vi "FlatSequence.vi"() -> ()   [LabVIEW 2015]
panel:
  in  "stop":bool
  in  "Tab Control":enum32{"Page 1", "Page 2", "Page 3"}(tab)
  in  "Slide":dbl(slide) scale=0.0..10.0
  out "String":string="Valor de Temperatura"
  out "Slide 2":dbl(slide) scale=0.0..10.0
  out "String 2":string="Agregacion de Parametros"
  out "String 3":string="Termina Proceso"
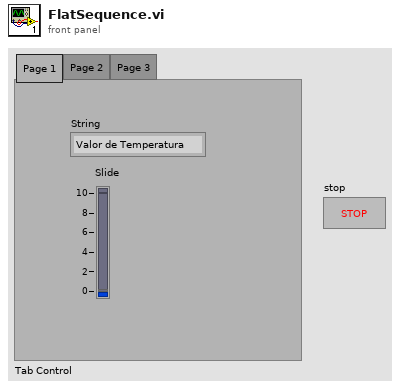
[diagram p1: front panel]
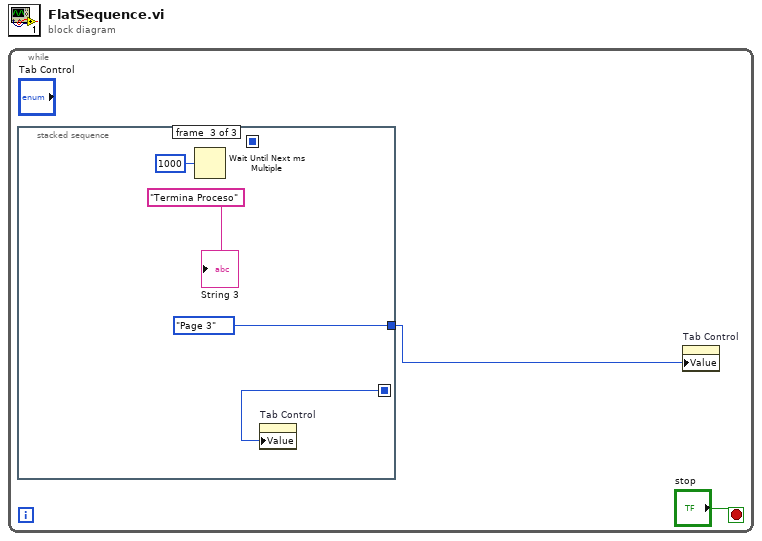
[diagram p0: block diagram]
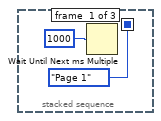
[diagram p2: hidden frame]
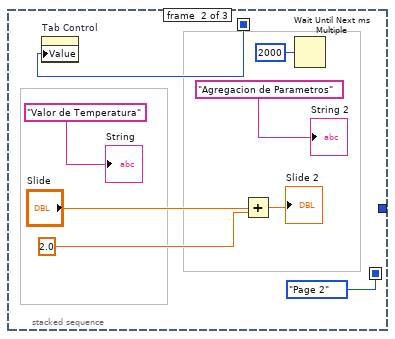
[diagram p3: hidden frame]
diagram:
  n1 = while {
    stop <- "stop" stop-if-true
    n2 = stacked-sequence {
      seq-local: [enum32{"Page 1", "Page 2", "Page 3"}."Page 1" ("Tab Control") _ _] -> [_ w6 _]
      seq-local: [_ enum32{"Page 1", "Page 2", "Page 3"}."Page 2" ("Tab Control") _] -> [_ _ w14]
      tunnel: [_ _ enum32{"Page 1", "Page 2", "Page 3"}."Page 3" ("Tab Control")] -> w2
      frame #0 {
        n3 = Wait Until Next ms Multiple(millisecond multiple=u32 1000) -> ()  [unwired: 1 out]
      }
      frame #1 {
        n4 = property on="Tab Control" class="TabCtl (strict)"("Value"=w6) -> ()  [unwired: 2 in, 2 out]
        n5 = Add(x="Slide", y=2.0) -> (x+y=→"Slide 2":dbl)
        n6 = Wait Until Next ms Multiple(millisecond multiple=u32 2000) -> ()  [unwired: 1 out]
        "String" <- "Valor de Temperatura"
        "String 2" <- "Agregacion de Parametros"
      }
      frame #2 {
        n7 = Wait Until Next ms Multiple(millisecond multiple=u32 1000) -> ()  [unwired: 1 out]
        n8 = property on="Tab Control" class="TabCtl (strict)"("Value"=w14) -> ()  [unwired: 2 in, 2 out]
        "String 3" <- "Termina Proceso"
      }
    }
    n9 = property on="Tab Control" class="TabCtl (strict)"("Value"=w2) -> ()  [unwired: 2 in, 2 out]
  }
